vi "Connect Bool.vi"(8 "Error In":errorcluster, 10 "Signal":string, 11 "Sender In":refnum<class "LQObject.lvclass">) -> (0 "Error Out":errorcluster, 2 "Bool Signal":refnum<user-event>, 3 "Sender Out":refnum<class "LQObject.lvclass">)   [LabVIEW 2013, in "Template.lvlib" / "LQCoreEngine.lvclass"]
uses:
  LQCoreEngine.lvclass
  LQObject/LQObject.lvclass
  LQIdentity/LQIdentity.lvclass/LQIdentity.ctl
  Connection Action.ctl
  Template.lvlib
  LQIdentity/LQIdentity.lvclass
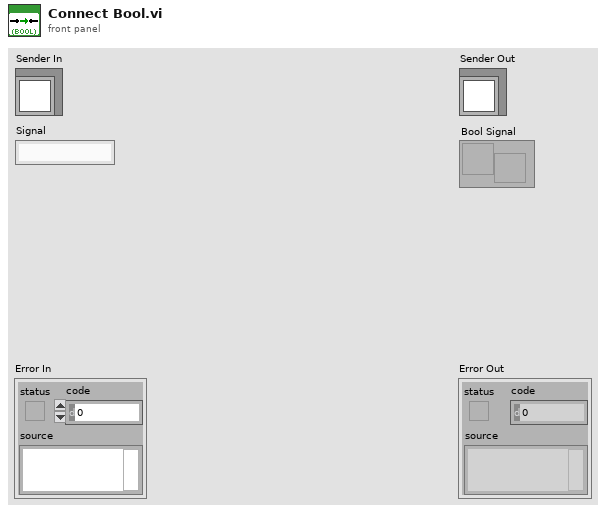
[diagram p1: front panel]
types:
  T1 = typedef "Template.lvlib/LQCoreEngine.lvclass/Connection Action.ctl" = enum16{"Init", "Add Connection", "Get Connections", "Clean Up"}
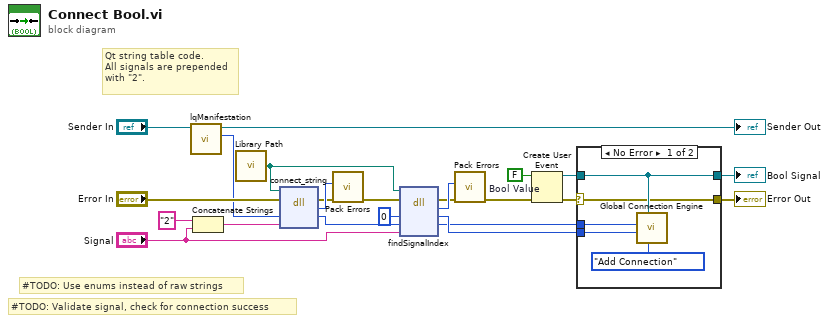
[diagram p0: block diagram]
diagram:
  w2 = FALSE  # Bool Value
  # "#TODO: Validate signal, check for connection success"
  # "Qt string table code.\nAll signals are prepended\nwith \"2\"."
  # "#TODO: Use enums instead of raw strings"
  n1 = call "lqManifestation.vi"("LQIdentity in"="Sender In") -> ("Manifestation"=w18:u64, "LQIdentity out"=→"Sender Out":refnum<class "LQObject.lvclass">)  [unwired: 9 in]
  n2 = Concatenate Strings("2" ("string"), "Signal") -> (w15:string)
  n3 = call "Library Path.vi"() -> ("Library Path"=w5:path)
  n4 = dll-call lib="?" fn="connect_string"(path in=w5, error in="Error In", "_instance"=w18, "encodedSignal"=w15) -> (error out=w10:errorcluster, "errorCode"=w11:i32, "_instance"=w17:u64)  [unwired: 2 in, 1 out]
  n5 = call "Pack Errors.vi"("Error In"=w10, "Error Code"=w11) -> ("Error Out"=w9:errorcluster)  [unwired: 9 in]
  n6 = dll-call lib="?" fn="findSignalIndex"(path in=w5, error in=w9, "retVal"=i64 0, "_instance"=w17, "encodedSignal"="Signal") -> (error out=w7:errorcluster, "errorCode"=w8:i32, "retVal"=w13:i64, "_instance"=w12:u64)  [unwired: 2 in, 1 out]
  n7 = call "Pack Errors.vi"("Error In"=w7, "Error Code"=w8) -> ("Error Out"=w6:errorcluster)  [unwired: 9 in]
  n8 = Create User Event(user event datatype=w2, error in=w6) -> (user event=w19:refnum<user-event>, error out=w4:errorcluster)
  n9 = case shown="No Error" w4 {
    selector: w4 -> [w24 w29]
    tunnel: w19 -> [w25 w30]
    tunnel: w13 -> [w28 _]
    tunnel: w12 -> [w27 _]
    tunnel: [w25 w30] -> w1
    tunnel: [w24 w29] -> w3
    frame No Error {
      n10 = call "Global Connection Engine.vi"("Connection Action"=Connection_Action."Add Connection", "Signal Channel"=w25, "Signal Index"=w28, "QObject Refnum"=w27) -> ()  [unwired: 7 in, 1 out]
    }
    frame Error {
    }
  }
  "Error Out" <- w3
  "Bool Signal" <- w1
